vi "BtnCtrl_Review(SubVI).vi"(8 "ButtonControlArray":refnum<vi>[](array[refnum]), 10 "RanFilenames":string[](array[string]), 11 "connection reference":T1) -> (3 "connection reference out":T1)   [LabVIEW 2013]
uses:
  <vilib>/addons/database/Connection.llb/Conn ObjectReference.ctl
  FYP_LabviewGlobal(SubVI).vi
  <vilib>/addons/database/_DB Variant To Data/Database Variant To Data.xnode
  <vilib>/addons/database/NI_Database_API.lvlib
panel:
  out "ScoredQuestionNo":string[](array[string])
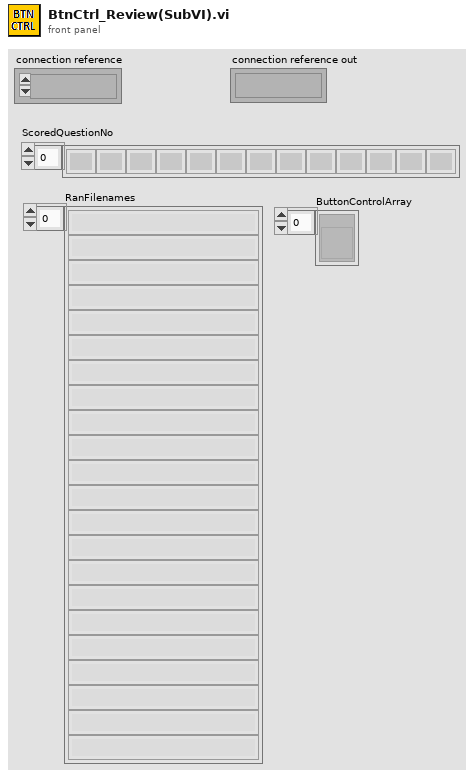
[diagram p1: front panel]
types:
  T1 = typedef "NI_Database_API.lvlib/Conn ObjectReference.ctl" = refnum<k1>
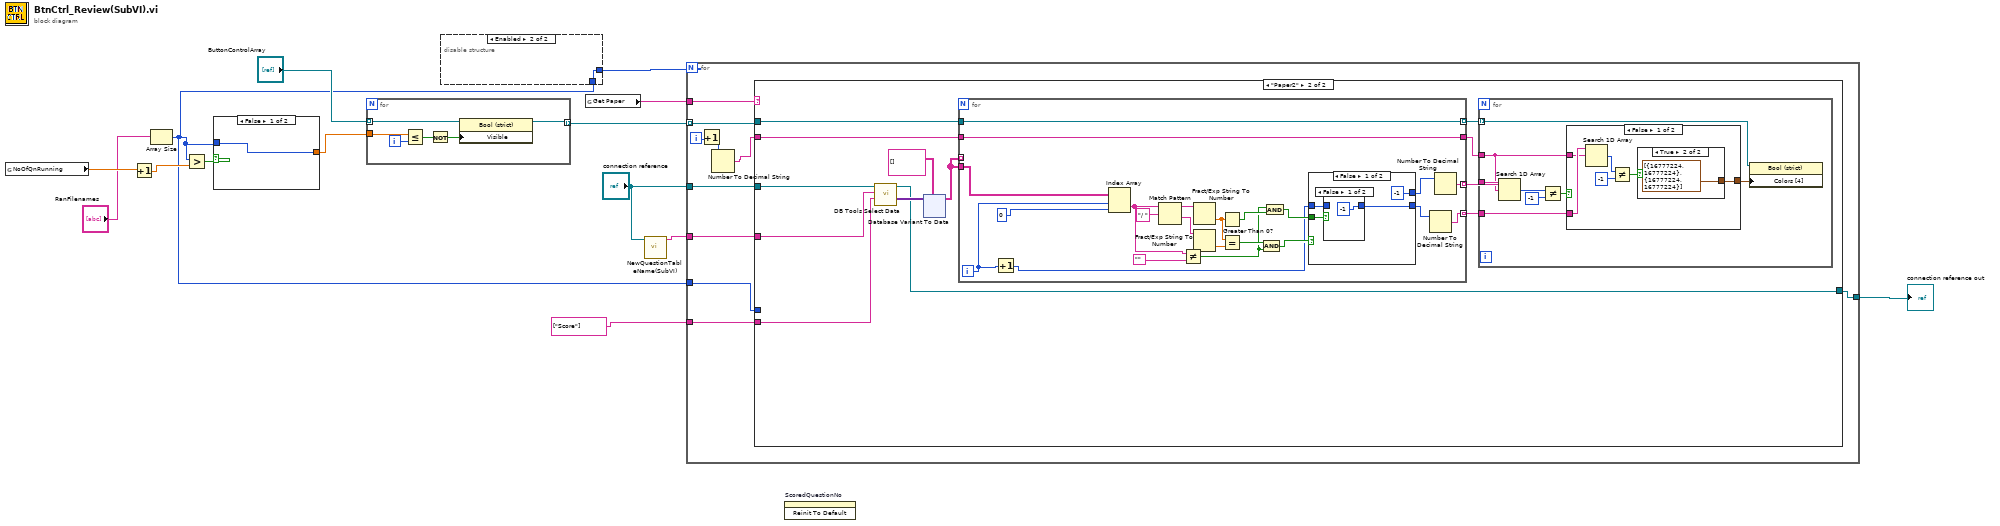
[diagram p0: block diagram]
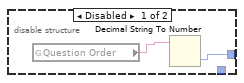
[diagram p2: hidden frame]
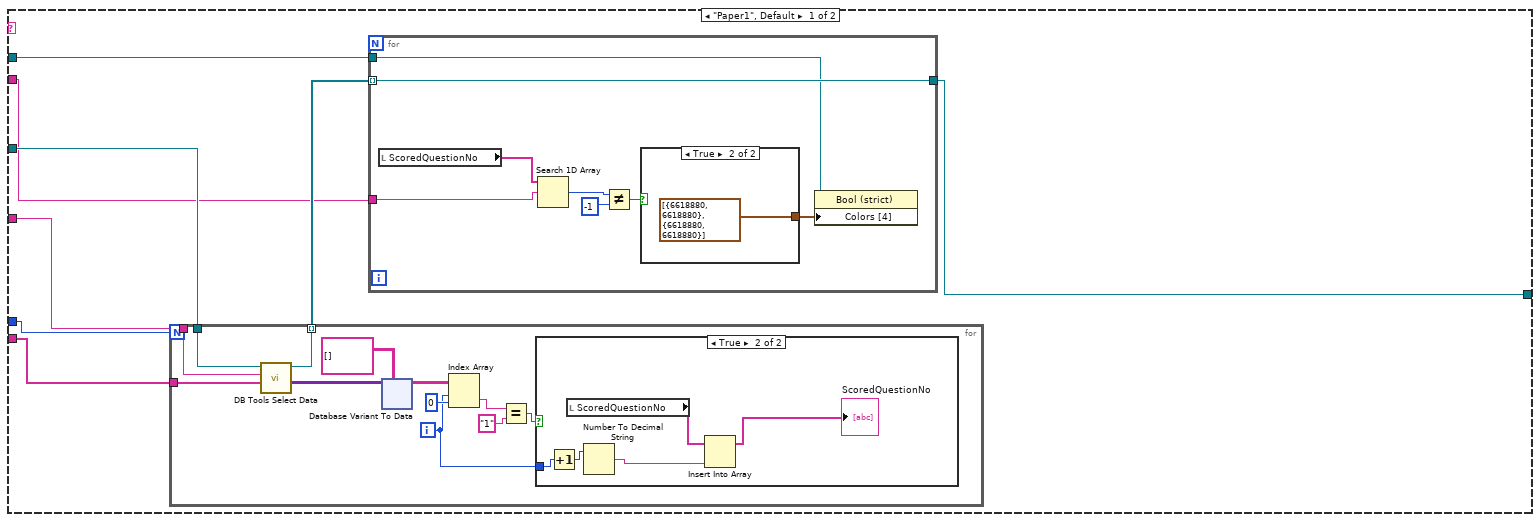
[diagram p3: hidden frame]
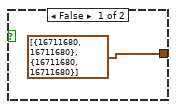
[diagram p5: hidden frame]
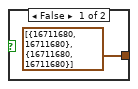
[diagram p6: hidden frame]
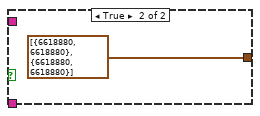
[diagram p7: hidden frame]
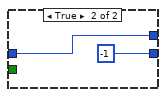
[diagram p9: hidden frame]
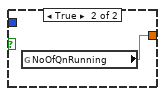
[diagram p10: hidden frame]
diagram:
  n1 = global read "FYP_LabviewGlobal(SubVI).vi" "NoOfQnRunning"() -> (w8:dbl)
  n2 = Increment(x=w8) -> (x+1=w7:dbl)
  n3 = Array Size(array="RanFilenames") -> (size(s)=w4:i32)
  n4 = Greater?(x=w4, y=w7) -> (0:w12:bool)
  n5 = case shown="False" w12 {
    tunnel: [w15 w16] -> w9
    tunnel: w4 -> [w15 _]
    frame False {
    }
    frame True {
      n6 = global read "FYP_LabviewGlobal(SubVI).vi" "NoOfQnRunning"() -> (w16:dbl)
    }
  }
  n7 = for {
    tunnel: w9 -> [w21]
    tunnel: "ButtonControlArray" -> [w22] mode=indexing
    tunnel: [w17] -> w13 mode=indexing
    i -> [w20]
    n8 = Less Or Equal?(x=w21, y=w20) -> (x <= y?=w19:bool)
    n9 = Not(x=w19) -> (.not. x?=w18:bool)
    n10 = property class="Bool (strict)"(reference=w22, "Visible"=w18) -> (reference out=w17:refnum<vi>)  [unwired: 1 in, 1 out]
  }
  n11 = disable-structure shown="Enabled" {
    disable-tunnel: [w23 w25] -> w5
    disable-tunnel: w4 -> [_ w25]
    frame Disabled {
      n12 = global read "FYP_LabviewGlobal(SubVI).vi" "Question Order"() -> (w24:string)
      n13 = Decimal String To Number(string=w24) -> (number=w23:i32)  [unwired: 2 in, 1 out]
    }
    frame Enabled {
    }
  }
  n14 = global read "FYP_LabviewGlobal(SubVI).vi" "Get Paper"() -> (w10:string)
  n15 = call "NewQuestionTableName(SubVI).vi"("connection reference"="connection reference") -> ("String"=w3:string)  [unwired: 9 in, 1 out]
  n16 = for {
    N: w5 -> [_]
    tunnel: w13 -> [w35] mode=indexing
    tunnel: "connection reference" -> [w34]
    tunnel: [w33] -> w11
    tunnel: w3 -> [w32]
    tunnel: w10 -> [w31]
    tunnel: string[] ["Score"] -> [w30]
    tunnel: w4 -> [w29]
    i -> [w27]
    n17 = Increment(x=w27) -> (x+1=w26:i32)
    n18 = Number To Decimal String(number=w26) -> (decimal integer string=w28:string)  [unwired: 1 in]
    n19 = case shown="\"Paper2\"" w31 {
      tunnel: w32 -> [w43 w127]
      tunnel: w34 -> [w42 w124]
      tunnel: [w40 w123] -> w33
      tunnel: w28 -> [w39 w120]
      tunnel: w35 -> [w38 w121]
      tunnel: w30 -> [w37 w115]
      tunnel: w29 -> [w36 _]
      frame "Paper1", Default {
        n20 = for {
          N: w36 -> [_]
          tunnel: w43 -> [w55]
          tunnel: w42 -> [w52]
          tunnel: [w51] -> w41 mode=indexing
          tunnel: w37 -> [w49]
          i -> [w45]
          n21 = call <vilib>:"DB Tools Select Data.vi"("columns"=w49, "table"=w55, "connection reference"=w52) -> ("data"=w54:variant[][], "connection reference out"=w51:T1)  [unwired: 3 in, 1 out]
          n22 = xnode "Database Variant To Data"("database variant"=w54, "type"=string[][] []) -> ("data"=w50:string[][])  [unwired: 1 in, 1 out]
          n23 = Index Array(array=w50, index (row)=w45, index (col)=0 ("disabled index (col)")) -> (element=w47:string)
          n24 = Equal?(x=w47, y="1") -> (x = y?=w46:bool)
          n25 = case shown="True" w46 {
            tunnel: w45 -> [_ w57]
            frame False {
            }
            frame True {
              n26 = Increment(x=w57) -> (x+1=w56:i32)
              n27 = local read "ScoredQuestionNo"() -> (w60:string[])
              n28 = Number To Decimal String(number=w56) -> (decimal integer string=w58:string)  [unwired: 1 in]
              n29 = Insert Into Array(array=w60, new element=w58) -> (→"ScoredQuestionNo":string[])  [unwired: 1 in]
            }
          }
        }
        n30 = for {
          tunnel: w41 -> [w110] mode=indexing
          tunnel: [w110] -> w40
          tunnel: w38 -> [w107]
          tunnel: w39 -> [w108]
          n31 = local read "ScoredQuestionNo"() -> (w105:string[])
          n32 = Search 1D Array(1D array=w105, element=w108) -> (index of element=w109:i32)  [unwired: 1 in]
          n33 = Not Equal?(x=w109, y=-1) -> (x != y?=w111:bool)
          n34 = case shown="True" w111 {
            tunnel: [cluster{u32, u32}[] [{16711680, 16711680}, {16711680, 16711680}] ("Colors [4]") cluster{u32, u32}[] [{6618880, 6618880}, {6618880, 6618880}] ("Colors [4]")] -> w106
            frame False {
            }
            frame True {
            }
          }
          n35 = property class="Bool (strict)"(reference=w107, "Colors [4]"=w106) -> ()  [unwired: 1 in, 2 out]
        }
      }
      frame "Paper2" {
        n36 = call <vilib>:"DB Tools Select Data.vi"("columns"=w115, "table"=w127, "connection reference"=w124) -> ("data"=w126:variant[][], "connection reference out"=w123:T1)  [unwired: 3 in, 1 out]
        n37 = xnode "Database Variant To Data"("database variant"=w126, "type"=string[][] []) -> ("data"=w122:string[][])  [unwired: 1 in, 1 out]
        n38 = for {
          tunnel: w122 -> [w158]
          tunnel: w122 -> [_] mode=indexing
          tunnel: w121 -> [w159]
          tunnel: w120 -> [w160]
          tunnel: [w156] -> w117 mode=indexing
          tunnel: [w154] -> w116 mode=indexing
          tunnel: [w160] -> w119
          tunnel: [w159] -> w118 mode=indexing
          i -> [w146]
          n39 = Increment(x=w146) -> (x+1=w145:i32)
          n40 = Index Array(array=w158, index (row)=w146, index (col)=0 ("disabled index (col)")) -> (element=w147:string)
          n41 = Match Pattern(string=w147, regular expression="/ ") -> (before substring=w164:string, after substring=w163:string)  [unwired: 1 in, 2 out]
          n42 = Not Equal?(x=w147, y="") -> (x != y?=w148:bool)
          n43 = Fract/Exp String To Number(string=w164) -> (number=w162:dbl)  [unwired: 3 in, 1 out]
          n44 = Fract/Exp String To Number(string=w163) -> (number=w161:dbl)  [unwired: 3 in, 1 out]
          n45 = Greater Than 0?(x=w162) -> (x > 0?=w150:bool)
          n46 = Equal?(x=w162, y=w161) -> (x = y?=w152:bool)
          n47 = And(x=w152, y=w148) -> (x .and. y?=w151:bool)
          n48 = And(x=w148, y=w150) -> (x .and. y?=w149:bool)
          n49 = case shown="False" w151 {
            tunnel: [-1 w174] -> w157
            tunnel: w145 -> [w169 w174]
            tunnel: w149 -> [w170 _]
            tunnel: [w167 -1] -> w155
            frame False {
              n50 = case shown="False" w170 {
                tunnel: [-1 w172] -> w167
                tunnel: w169 -> [_ w172]
                frame False {
                }
                frame True {
                }
              }
            }
            frame True {
            }
          }
          n51 = Number To Decimal String(number=w155) -> (decimal integer string=w154:string)  [unwired: 1 in]
          n52 = Number To Decimal String(number=w157) -> (decimal integer string=w156:string)  [unwired: 1 in]
        }
        n53 = for {
          tunnel: w119 -> [w128]
          tunnel: w117 -> [w129]
          tunnel: w118 -> [w131] mode=indexing
          tunnel: w116 -> [w130]
          n54 = Search 1D Array(1D array=w129, element=w128) -> (index of element=w133:i32)  [unwired: 1 in]
          n55 = Not Equal?(x=w133, y=-1) -> (x != y?=w134:bool)
          n56 = case shown="False" w134 {
            tunnel: [w138 cluster{u32, u32}[] [{6618880, 6618880}, {6618880, 6618880}] ("Colors [4]")] -> w135
            tunnel: w130 -> [w137 _]
            tunnel: w128 -> [w136 _]
            frame False {
              n57 = Search 1D Array(1D array=w137, element=w136) -> (index of element=w140:i32)  [unwired: 1 in]
              n58 = Not Equal?(x=w140, y=-1) -> (x != y?=w139:bool)
              n59 = case shown="True" w139 {
                tunnel: [cluster{u32, u32}[] [{16711680, 16711680}, {16711680, 16711680}] ("Colors [4]") cluster{u32, u32}[] [{16777224, 16777224}, {16777224, 16777224}] ("Colors [4]")] -> w138
                frame False {
                }
                frame True {
                }
              }
            }
            frame True {
            }
          }
          n60 = property class="Bool (strict)"(reference=w131, "Colors [4]"=w135) -> ()  [unwired: 1 in, 2 out]
        }
      }
    }
  }
  "connection reference out" <- w11
  n61 = invoke on="ScoredQuestionNo" class="Arr (strict)" method="Reinit To Default"() -> ()  [unwired: 3 in, 3 out]
